vi "Calculate Rate.vi"(10 "# of Pts":dbl, 11 "Data In":T1[](array[typedef])) -> (0 "Value":dbl, 1 "residue":dbl, 2 "slope":dbl, 3 "Data Out":T1[](array[typedef]), 4 "Time":dbl)   [LabVIEW 2018]
uses:
  Pressure Point.ctl
  <vilib>/Analysis/6fits.llb/Curve Fitting Criteria.ctl
  <vilib>/Analysis/NI_AALPro.lvlib
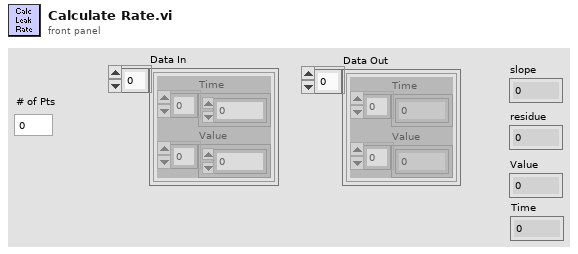
[diagram p1: front panel]
types:
  T1 = typedef "Pressure Point.ctl" = cluster{"Time":dbl[], "Value":dbl[]}
  T2 = typedef "NI_AALPro.lvlib/Curve Fitting Criteria.ctl" = u16
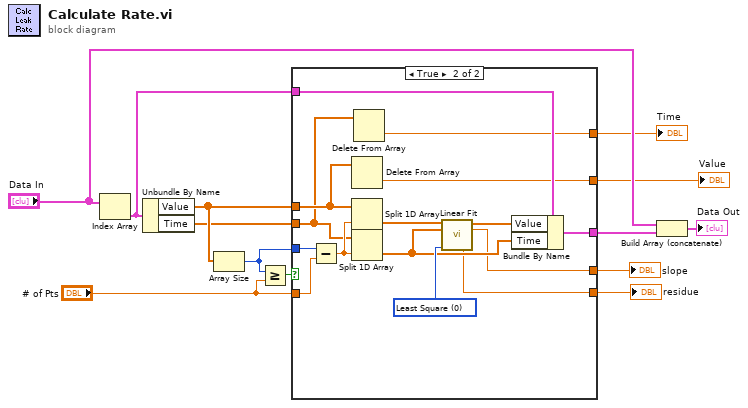
[diagram p0: block diagram]
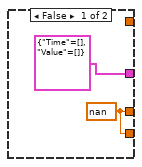
[diagram p2: hidden frame]
diagram:
  n1 = Index Array(array="Data In") -> (element=w8:T1)  [unwired: 1 in]
  n2 = Unbundle By Name(w8) -> ("Value"=w12:dbl[], "Time"=w11:dbl[])
  n3 = Array Size(array=w12) -> (size(s)=w10:i32)
  n4 = Greater Or Equal?(x=w10, y="# of Pts") -> (x >= y?=w13:bool)
  n5 = case shown="True" w13 {
    tunnel: w12 -> [_ w19]
    tunnel: w11 -> [_ w17]
    tunnel: w10 -> [_ w30]
    tunnel: "# of Pts" -> [_ w29]
    tunnel: w8 -> [_ w25]
    tunnel: [T1 {"Time"=[], "Value"=[]} ("output cluster") w22] -> w7
    tunnel: [w15 w21] -> w6
    tunnel: [w15 w20] -> w5
    tunnel: [_ w18] -> w1
    tunnel: [_ w16] -> w2
    frame False {
      w15 = nan ("slope")
    }
    frame True {
      w26 = T2 0 items=["Least Square", "Least Absolute Residual", "Bisquare"] ("method")
      n6 = Subtract(x=w30, y=w29) -> (x-y=w28:dbl)
      n7 = Delete From Array(array=w19) -> (deleted portion=w18:dbl)  [unwired: 2 in, 1 out]
      n8 = Split 1D Array(array=w19, index=w28) -> (second subarray=w27:dbl[])  [unwired: 1 out]
      n9 = Split 1D Array(array=w17, index=w28) -> (second subarray=w23:dbl[])  [unwired: 1 out]
      n10 = Delete From Array(array=w17) -> (deleted portion=w16:dbl)  [unwired: 2 in, 1 out]
      n11 = call <vilib>:"Linear Fit.vi"("Y"=w27, "X"=w23, "method"=w26) -> ("Best Linear Fit"=w24:dbl[], "slope"=w21:dbl, "residue"=w20:dbl)  [unwired: 8 in, 2 out]
      n12 = Bundle By Name(cluster=w25, "Value"=w24, "Time"=w23) -> (w22:T1)
    }
  }
  "slope" <- w6
  "residue" <- w5
  "Value" <- w1
  "Time" <- w2
  n13 = Build Array (concatenate)("Data In", w7) -> (→"Data Out":T1[])
